vi "12_11_Fxp_addation.vi"(1 "y":fxp<+/-,11,12>, 2 "x":fxp<+/-,11,12>) -> (0 "x+y":fxp<+/-,11,12>)   [LabVIEW 2020]
panel:
  in  "x 2":fxp<+/-,11,12>
  out "x+y 2":fxp<+/-,11,12>
  in  "y 2":fxp<+/-,11,12>
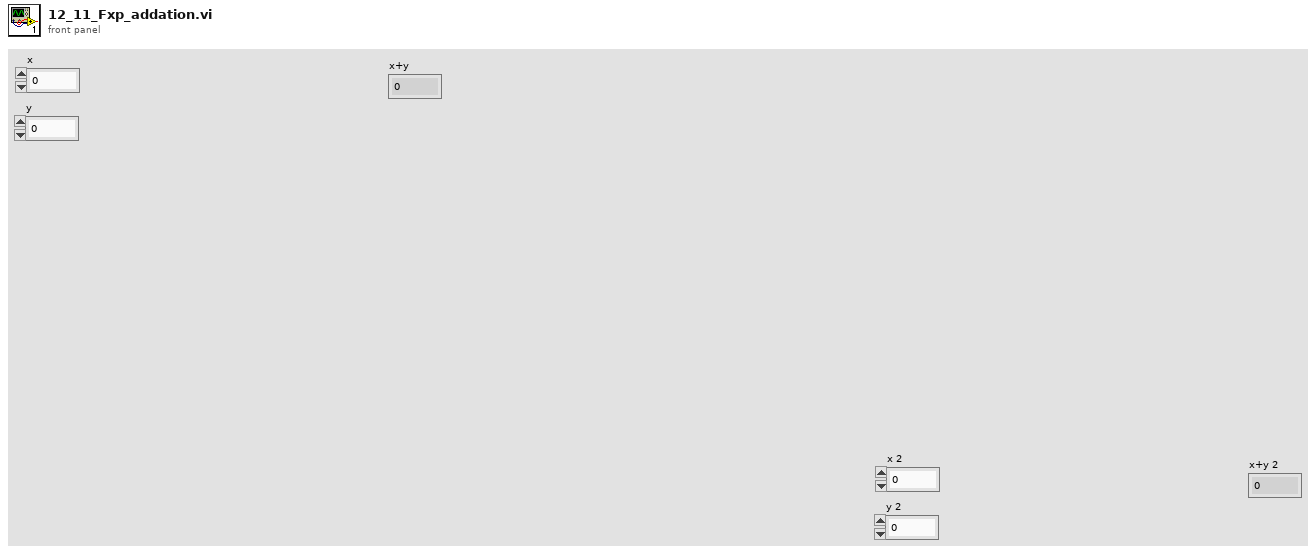
[diagram p1: front panel]
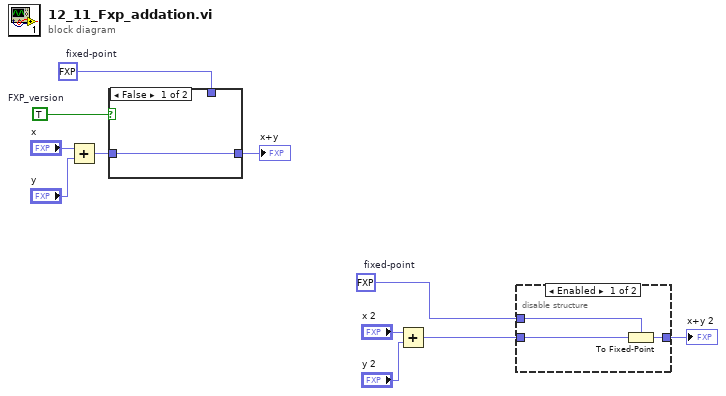
[diagram p0: block diagram]
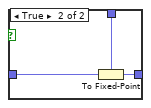
[diagram p3: hidden frame]
diagram:
  w1 = fxp<+/-,11,12> 0.0  # fixed-point
  w6 = fxp<+/-,11,12> 0.0  # fixed-point
  w7 = TRUE  # FXP_version
  n1 = Add(x="x", y="y") -> (x+y=w8:fxp<+/-,12,13>)
  n2 = case shown="False" w7 {
    tunnel: [w12 w15] -> w9
    tunnel: w8 -> [w12 w14]
    tunnel: w6 -> [_ w13]
    frame False {
    }
    frame True {
      n3 = To Fixed-Point(fixed-point type=w13, number=w14) -> (fixed-point=w15:fxp<+/-,11,12>)
    }
  }
  "x+y" <- w9
  n4 = Add(x="x 2", y="y 2") -> (x+y=w2:fxp<+/-,12,13>)
  n5 = disable-structure shown="Enabled" {
    disable-tunnel: [w18 w19] -> w3
    disable-tunnel: w2 -> [w17 w19]
    disable-tunnel: w1 -> [w16 _]
    frame Enabled {
      n6 = To Fixed-Point(fixed-point type=w16, number=w17) -> (fixed-point=w18:fxp<+/-,11,12>)
    }
    frame Disabled {
    }
  }
  "x+y 2" <- w3
